vi "testOutputDOF.vi"(8 "error in (no error)":errorcluster) -> (0 "error out":errorcluster)   [LabVIEW 2016]
doc: "Test the setStateToState0.vi. This test considers the state and state0."
uses:
  ZTAAC/ZTAAC.lvclass
  StrictDef/DofGroup.ctl
  StrictDef/InstName.ctl
  <vilib>/addons/_JKI Toolkits/Caraya/classes/Test/Test.lvclass
  <vilib>/addons/_JKI Toolkits/Caraya/classes/Assert/Assert.lvclass
panel:
  in  "ZTAAC.lvclass":refnum<class "ZTAAC.lvclass">
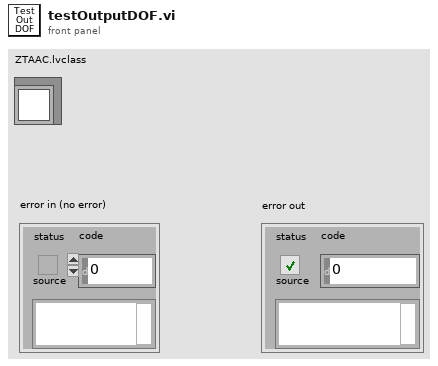
[diagram p1: front panel]
types:
  T1 = typedef "InstName.ctl" = enum16{"lsst", "comcam"}
  T2 = cluster{"Config Dir":path, "Inst Name":T1, "OptStateEsti Config File Name":string, "Mapping File Name":string, "Wavelength Table":string, "Intrinc Zk File Name":string, "y2 Corection File Name":string, "Index DOF File Name":string, "OptCtrl Config File Name":string, "State 0 File Name":string, "Weighting File Name":string, "PSSN Alpha File Name":string, "Authority Files":cluster{"Rigid Body Stroke File":string, "M1M3 Subsystem":cluster{"Mirror":string, "Actuatro Force File":string}, "M2 Subsystem":cluster{"Mirror":string, "Actuatro Force File":string}, "Num of Bending Mode":i32}, "Truncation Threshold":dbl}
  T3 = typedef "DofGroup.ctl" = enum16{"M2 Hex Pos", "Cam Hex Pos", "M1M3 Bend", "M2 Bend"}
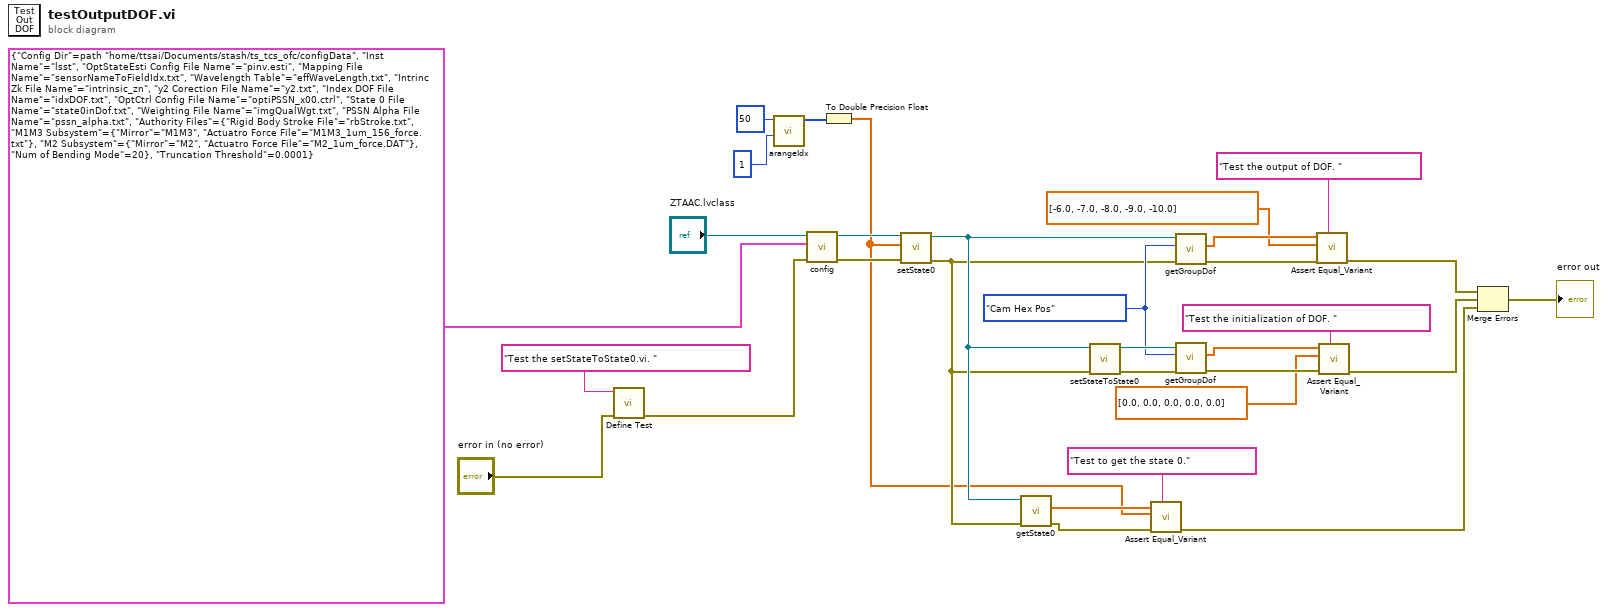
[diagram p0: block diagram]
diagram:
  w25 = DofGroup."Cam Hex Pos" ("DOF Group")
  n1 = call <vilib>:"Define Test.vi"("error in (no error)"="error in (no error)", "Label (VI Title)"="Test the setStateToState0.vi. ") -> ("error out"=w24:errorcluster)  [unwired: 9 in]
  n2 = call "arangeIdx.vi"("Offset"=1, "Number"=50) -> ("Idx Array"=w28:i32[])  [unwired: 9 in]
  n3 = call "config.vi"("error in (no error)"=w24, "ZTAAC Configuration"=T2 {"Config Dir"=path "/home/ttsai/Documents/stash/ts_tcs_ofc/configData", "Inst Name"=enum."lsst", "OptStateEsti Config File Name"="pinv.esti", "Mapping File Name"="sensorNameToFieldIdx.txt", "Wavelength Table"="effWaveLength.txt", "Intrinc Zk File Name"="intrinsic_zn", "y2 Corection File Name"="y2.txt", "Index DOF File Name"="idxDOF.txt", "OptCtrl Config File Name"="optiPSSN_x00.ctrl", "State 0 File Name"="state0inDof.txt", "Weighting File Name"="imgQualWgt.txt", "PSSN Alpha File Name"="pssn_alpha.txt", "Authority Files"={"Rigid Body Stroke File"="rbStroke.txt", "M1M3 Subsystem"={"Mirror"="M1M3", "Actuatro Force File"="M1M3_1um_156_force.txt"}, "M2 Subsystem"={"Mirror"="M2", "Actuatro Force File"="M2_1um_force.DAT"}, "Num of Bending Mode"=20}, "Truncation Threshold"=0.0001}, "ZTAAC in"="ZTAAC.lvclass") -> ("error out"=w21:errorcluster, "ZTAAC out"=w30:refnum<class "ZTAAC.lvclass">)  [unwired: 7 in]
  n4 = To Double Precision Float(number=w28) -> (double precision float=w3:dbl[])
  n5 = call "setState0.vi"("error in (no error)"=w21, "State 0 in DOF"=w3, "ZTAAC in"=w30) -> ("error out"=w7:errorcluster, "ZTAAC out"=w8:refnum<class "ZTAAC.lvclass">)  [unwired: 7 in]
  n6 = call-dynamic "getState0.vi"("error in (no error)"=w7, "ZTAAC in"=w8) -> ("error out"=w5:errorcluster, "State 0 in DOF"=w6:dbl[])  [unwired: 7 in, 1 out]
  n7 = call "setStateToState0.vi"("error in (no error)"=w7, "ZTAAC in"=w8) -> ("error out"=w20:errorcluster, "ZTAAC out"=w26:refnum<class "ZTAAC.lvclass">)  [unwired: 8 in]
  n8 = call <vilib>:"Assert Equal_Variant.vi"("Label"="Test to get the state 0.", "error in (no error)"=w5, "Y"=w3, "X"=w6) -> ("error out"=w4:errorcluster)  [unwired: 7 in]
  n9 = call "getGroupDof.vi"("error in (no error)"=w7, "DOF Group"=w25, "ZTAAC in"=w8) -> ("error out"=w19:errorcluster, "DOF"=w16:dbl[])  [unwired: 6 in, 1 out]
  n10 = call "getGroupDof.vi"("error in (no error)"=w20, "DOF Group"=w25, "ZTAAC in"=w26) -> ("error out"=w18:errorcluster, "DOF"=w17:dbl[])  [unwired: 6 in, 1 out]
  n11 = call <vilib>:"Assert Equal_Variant.vi"("Label"="Test the output of DOF. ", "error in (no error)"=w19, "Y"=dbl[] [-6.0, -7.0, -8.0, -9.0, -10.0], "X"=w16) -> ("error out"=w15:errorcluster)  [unwired: 7 in]
  n12 = call <vilib>:"Assert Equal_Variant.vi"("Label"="Test the initialization of DOF. ", "error in (no error)"=w18, "Y"=dbl[] [0.0, 0.0, 0.0, 0.0, 0.0], "X"=w17) -> ("error out"=w14:errorcluster)  [unwired: 7 in]
  n13 = Merge Errors(w15, w14, w4) -> (→"error out":errorcluster)
